vi "CTRnode.vi"(8 "error in":errorcluster) -> (0 "error out":errorcluster)   [LabVIEW 2024]
uses:
  Control/StreamTypeDef.ctl
  Control/streamIO_states.ctl
  <vilib>/Platform/TimedLoop/XDataNode/timing_clust.ctl
  <vilib>/Platform/TimedLoop/XDataNode/nitl_modes.ctl
  <vilib>/Platform/TimedLoop/XDataNode/wakeup.ctl
  <vilib>/Platform/TimedLoop/TimeConversion.llb/rt-milliseconds-to-rel-time.vi
  <vilib>/Platform/TimedLoop/TimeConversion.llb/rt-milliseconds-to-timestamp.vi
  <vilib>/platform/TimedLoop/XDataNode/XDataNode.xnode
  <vilib>/Platform/TimedLoop/XDataNode/XDNodeRunTimeDep.lvlib
panel:
  out "Logging Clock (ms)":cluster{"Period":i64, i64}(graph)
  in  "stop":bool
  out "Streaming Clock (ms)":cluster{dbl, "Period":dbl}(graph)
  in  "StreamTypeDef":T1
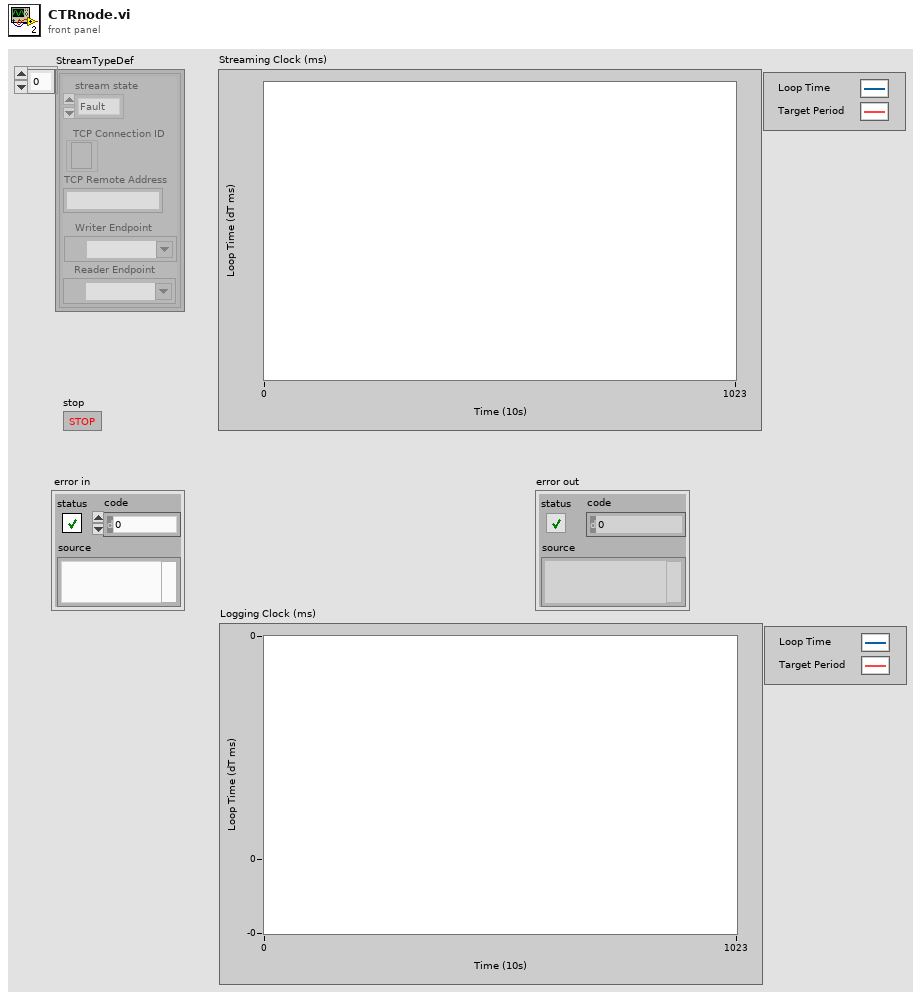
[diagram p1: front panel]
types:
  T1 = typedef "StreamTypeDef.ctl" = cluster{"stream state":T2, "TCP Remote Address":string, "TCP Connection ID":refnum<k5>, "Reader Endpoint":refnum<k21>, "Writer Endpoint":refnum<k21>}[]
  T2 = typedef "streamIO_states.ctl" = enum16{"Fault", "Initilize", "Stream", "Close"}
  T3 = cluster{"stream state":T2, "TCP Remote Address":string, "TCP Connection ID":refnum<k5>, "Reader Endpoint":refnum<k21>, "Writer Endpoint":refnum<k21>}
  T4 = typedef "XDNodeRunTimeDep.lvlib/timing_clust.ctl" = cluster{"Expected End [f-1]":u64, "Actual End [f-1]":u64, "Finished Late? [f-1]":bool, "Expected End [i-1]":u64, "Actual End [i-1]":u64, "Finished Late? [i-1]":bool, "Expected Start [i]":u64, "Actual Start [i]":u64, "Expected Start [f]":u64, "Actual Start [f]":u64, "Source Name":string, "Structure Name":string, "Period":i64, "Deadline":i64, "Offset":i64, "Start":i64, "Priority":i32, "Timeout":i32, "Mode":T5, "Wakeup Reason":T6, "Error":errorcluster, "Source Type":string, "Secondary Source Type":string, "Global End Time":u64, "Global Start Time":u64, "Frame Duration":u64, "Iteration Duration":u64, "Assigned CPU":i32, "I/O Scan Engine Mode":u32}
  T5 = typedef "XDNodeRunTimeDep.lvlib/nitl_modes.ctl" = enum32{"No Change", "Process missed periods, maintain original phase", "Discard missed periods, maintain original phase", "Process missed periods, ignore original phase", "Discard missed periods, ignore original phase"}
  T6 = typedef "XDNodeRunTimeDep.lvlib/wakeup.ctl" = enum32{"Normal", "Aborted", "Asynchronous wakeup", "Timing source error", "Timed loop error", "Timeout"}
  T7 = cluster{"stream state":T2, "TCP Remote Address":string, "TCP Connection ID":refnum<k5>, "Reader Endpoint":refnum<k21>, "Writer Endpoint":refnum<k21>}[]
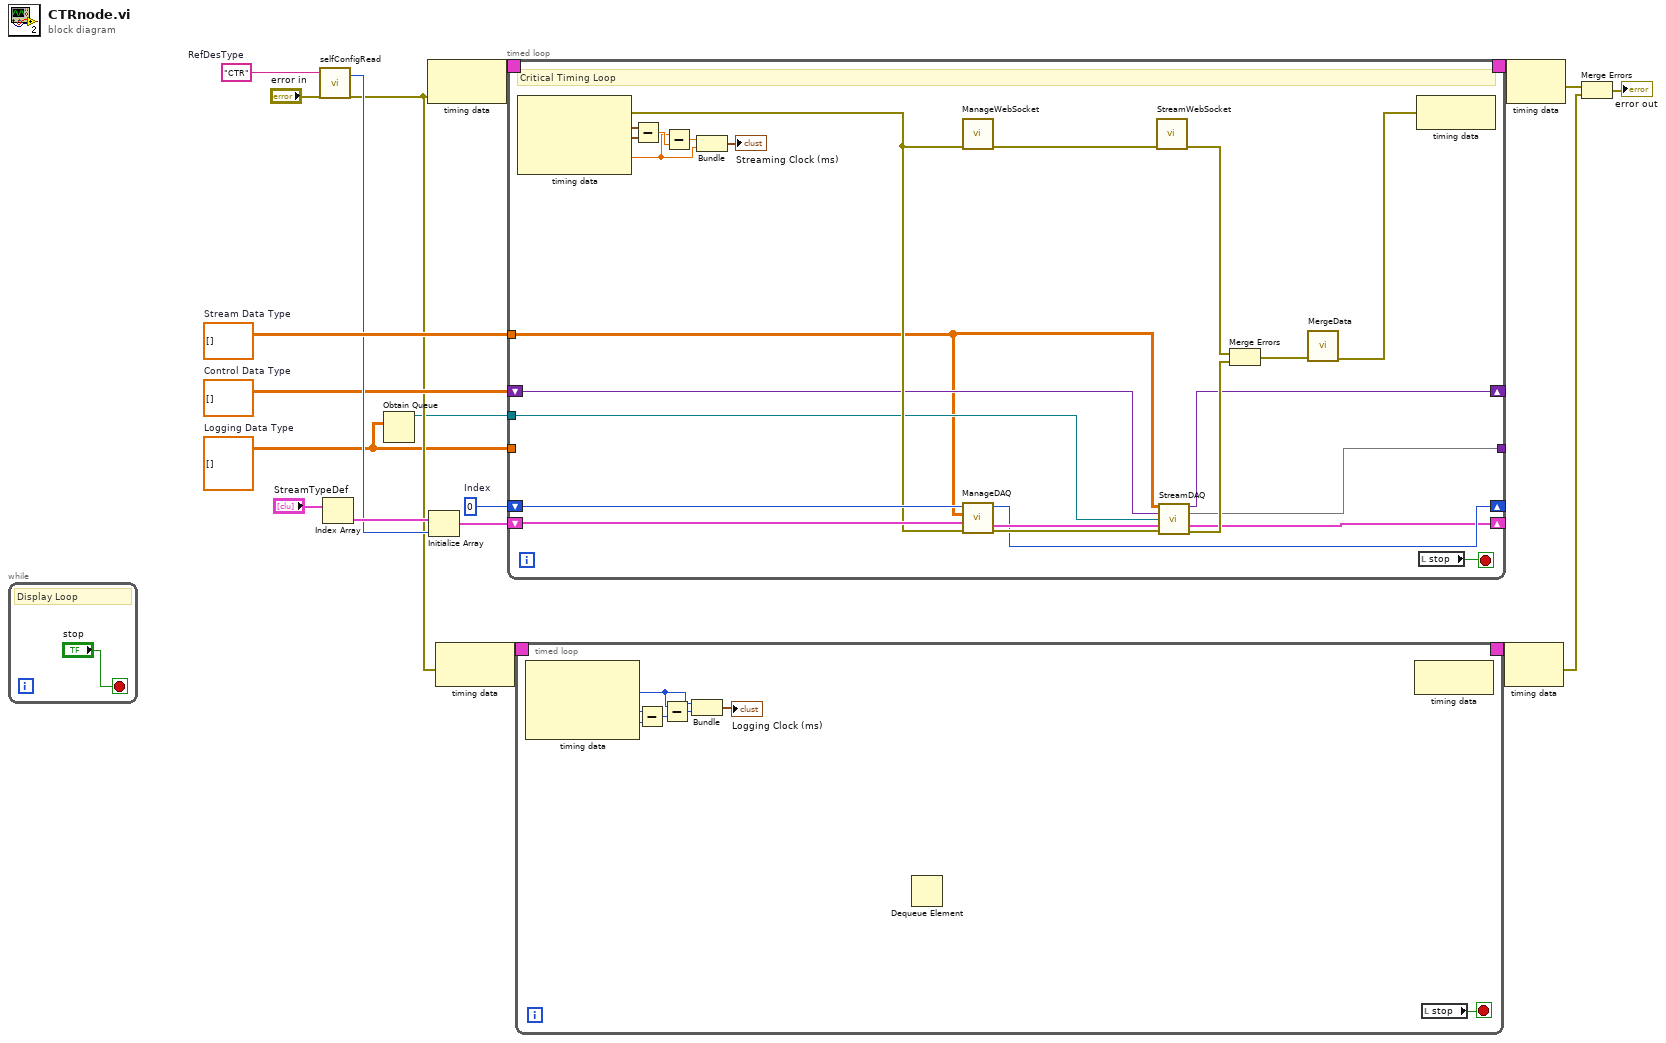
[diagram p0: block diagram]
diagram:
  w9 = dbl[][] []  # Control Data Type
  w2 = dbl[][][] []  # Logging Data Type
  w16 = "CTR"  # RefDesType
  w18 = dbl[][] []  # Stream Data Type
  w19 = 0  # Index
  n1 = while {
    stop <- "stop" stop-if-true
    # "Display Loop"
  }
  n2 = call "selfConfigRead.vi"("RefDesType"=w16, "error in"="error in") -> ("DAQ Node Count"=w12:i32, "error out"=w6:errorcluster)  [unwired: 13 in, 3 out]
  n3 = Index Array(array="StreamTypeDef") -> (element=w14:T3)  [unwired: 1 in]
  n4 = Obtain Queue(element data type=w2) -> (queue out=w1:refnum<queue>)  [unwired: 4 in, 2 out]
  n5 = node-c288(w6) -> (w11:T4)
  n6 = Initialize Array(w14, w12) -> (w13:T7)
  n7 = node-c288(w6) -> (w8:T4)
  n8 = timed-loop {
    timing: w11 -> [_]
    timing-out: [_] -> w10
    shift-right: [w35] -> _
    shift-left: w13 -> [w43]
    shift-right: [w36] -> _
    shift-left: w19 -> [w44]
    shift-right: [w25] -> _
    shift-left: w9 -> [w26]
    tunnel: w18 -> [w21]
    tunnel: w2 -> [_]
    tunnel: [w24] -> _
    tunnel: w1 -> [w22]
    stop <- w23 stop-if-true
    # "Critical Timing Loop"
    n9 = node-c288() -> (w34:errorcluster, w32:timestamp, w31:timestamp, w28:dbl)  [unwired: 1 in]
    n10 = Subtract(x=w32, y=w31) -> (x-y=w30:dbl)
    n11 = Subtract(x=w28, y=w30) -> (x-y=w29:dbl)
    n12 = Bundle(w29, "Period"=w28) -> (→"Streaming Clock (ms)":cluster{dbl, "Period":dbl})  [unwired: 1 in]
    n13 = call "ManageWebSocket.vi"("error in"=w34) -> ("error out"=w38:errorcluster)  [unwired: 10 in]
    n14 = call "ManageDAQ.vi"("error in"=w34, "StreamTypeDef"=w43, "data type"=w21, "index"=w44) -> ("error out"=w42:errorcluster, "StreamTypeDef"=w37:T1, "Index+1"=w36:i32)  [unwired: 5 in]
    n15 = call "StreamWebSocket.vi"("error in"=w38) -> ("error out"=w39:errorcluster)  [unwired: 10 in]
    n16 = call "StreamDAQ.vi"(0:w21, "control data type"=w26, "Logging Queue"=w22, "StreamTypeDef"=w37, "error in"=w42) -> ("control data out"=w25:variant, 6:w24, "StreamTypeDef"=w35:T1, "error out"=w40:errorcluster)  [unwired: 7 in]
    n17 = Merge Errors(w39, w40) -> (w41:errorcluster)
    n18 = call "MergeData.vi"("error in"=w41) -> ("error out"=w33:errorcluster)  [unwired: 10 in]
    n19 = node-c288(w33) -> ()  [unwired: 1 out]
    n20 = local read "stop"() -> (w23:bool)
  }
  n21 = timed-loop {
    timing: w8 -> [_]
    timing-out: [_] -> w7
    stop <- w56 stop-if-true
    n22 = node-c288() -> (w57:i64, w60:i64, w61:i64)  [unwired: 1 in, 1 out]
    n23 = Subtract(x=w60, y=w61) -> (x-y=w62:i64)
    n24 = Subtract(x=w57, y=w62) -> (x-y=w59:i64)
    n25 = Bundle("Period"=w57, w59) -> (→"Logging Clock (ms)":cluster{"Period":i64, i64})  [unwired: 1 in]
    n26 = Dequeue Element() -> ()  [unwired: 3 in, 4 out]
    n27 = node-c288() -> ()  [unwired: 1 in, 1 out]
    n28 = local read "stop"() -> (w56:bool)
  }
  n29 = node-c288(w7) -> (w3:errorcluster)
  n30 = node-c288(w10) -> (w4:errorcluster)
  n31 = Merge Errors(w4, w3) -> (→"error out":errorcluster)
